vi "Write Integer.vi"(8 "error in":errorcluster, 9 "Element:":i16, 10 "PLC Address":string="N7:0", 11 "IP Address:":string="192.168.100.15") -> (0 "error out":errorcluster)   [LabVIEW 2018]
uses:
  <vilib>/ethernetip/ethernetip.lvlib
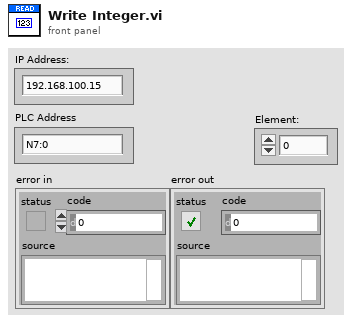
[diagram p1: front panel]
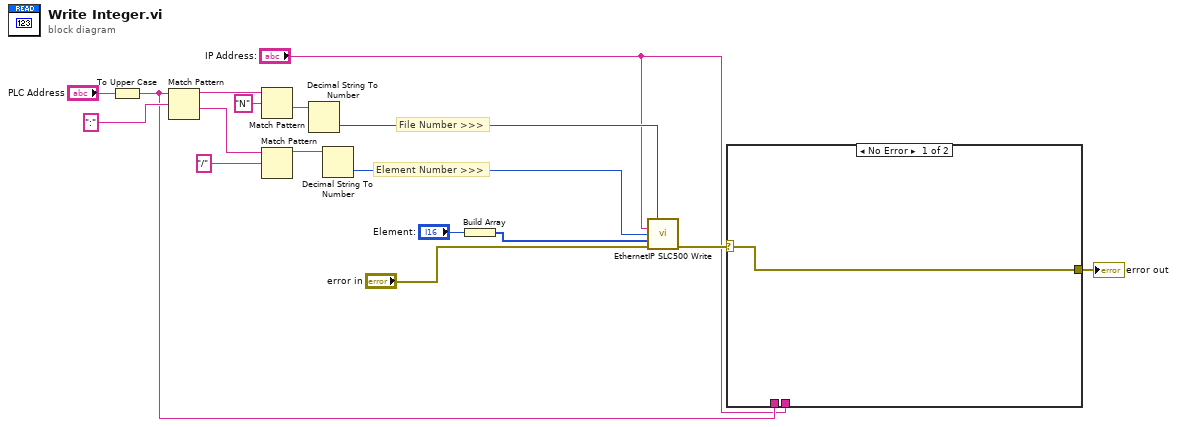
[diagram p0: block diagram]
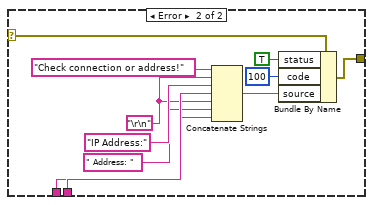
[diagram p2: hidden frame]
diagram:
  # "Element Number >>>"
  # "File Number >>>"
  n1 = To Upper Case(1:"PLC Address") -> (0:w4:string)
  n2 = Match Pattern(string=w4, regular expression=":") -> (before substring=w16:string, after substring=w11:string)  [unwired: 1 in, 2 out]
  n3 = Match Pattern(string=w16, regular expression="N") -> (after substring=w13:string)  [unwired: 1 in, 3 out]
  n4 = Match Pattern(string=w11, regular expression="/") -> (before substring=w9:string)  [unwired: 1 in, 3 out]
  n5 = Decimal String To Number(string=w13) -> (number=w12:i32)  [unwired: 2 in, 1 out]
  n6 = Decimal String To Number(string=w9) -> (number=w8:i32)  [unwired: 2 in, 1 out]
  n7 = Build Array("Element:") -> (w1:i16[])
  n8 = call-poly <vilib>:"EthernetIP SLC500 Write.vi"("File Number"=w12, "Network Path"="IP Address:", "Element Number"=w8, "Data"=w1, "error in"="error in") -> ("error out"=w6:errorcluster)  [unwired: 9 in, 1 out]
  n9 = case shown="No Error" w6 {
    selector: w6 -> [w18 w29]
    tunnel: [w18 w28] -> w5
    tunnel: w4 -> [_ w19]
    tunnel: "IP Address:" -> [_ w22]
    frame No Error {
    }
    frame Error {
      w21 = "\r\n"
      n10 = Concatenate Strings("Check connection or address!" ("source"), w21, "IP Address:", w22, w21, " Address: ", w19) -> (w23:string)
      n11 = Bundle By Name(cluster=w29, "status"=TRUE, "code"=100, "source"=w23) -> (w28:errorcluster)
    }
  }
  "error out" <- w5
